vi "Get Devices In Family.vi"(8 "Error In":errorcluster, 11 "Device Family":T4) -> (0 "Error Out":errorcluster, 3 "Devices":string[](array[string]))   [LabVIEW 2013, in "LVH-LINX.lvlib"]
uses:
  <vilib>/LabVIEW Hacker/LINX/LVH-LINX.lvlib
  <vilib>/LabVIEW Hacker/LINX/Private/Type Defs/Device Family.ctl
  <vilib>/LabVIEW Hacker/LINX/Private/Type Defs/Devices - Digilent.ctl
  <vilib>/LabVIEW Hacker/LINX/Private/Type Defs/Devices - NI.ctl
  <vilib>/LabVIEW Hacker/LINX/Private/Type Defs/Devices - Arduino.ctl
panel:
  in  "Arduino Device":T1
  in  "NI Device":T2
  in  "Digilent Device":T3
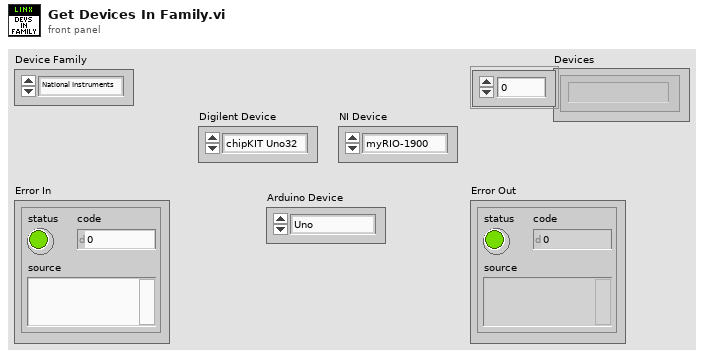
[diagram p1: front panel]
types:
  T1 = typedef "LVH-LINX.lvlib/Devices - Arduino.ctl" = enum16{"Uno", "Mega 2560", "Leonardo", "Due", "Yun", "Nano", "Pro Mini", "Pro", "Fio", "Mega1280"}
  T2 = typedef "LVH-LINX.lvlib/Devices - NI.ctl" = enum16{"myRIO-1900", "myRIO-1950"}
  T3 = typedef "LVH-LINX.lvlib/Devices - Digilent.ctl" = enum16{"chipKIT Uno32", "chipKIT uC32", "chipKIT Max32", "chipKIT WF32"}
  T4 = typedef "LVH-LINX.lvlib/Device Family.ctl" = enum8{"National Instruments", "Digilent", "Arduino"}
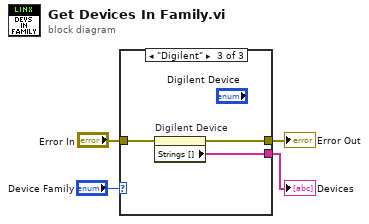
[diagram p0: block diagram]
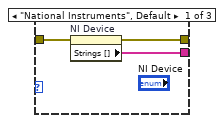
[diagram p2: hidden frame]
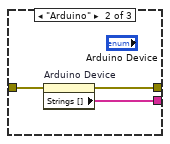
[diagram p3: hidden frame]
diagram:
  n1 = case shown="\"Digilent\"" "Device Family" {
    tunnel: "Error In" -> [w7 w9 w12]
    tunnel: [w5 w8 w13] -> w2
    tunnel: [w6 w10 w11] -> w1
    frame "National Instruments", Default {
      n2 = property on="NI Device" class="Enum (strict)"(error in=w7) -> (error out=w6:errorcluster, "Strings []"=w5:string[])  [unwired: 1 in, 1 out]
    }
    frame "Arduino" {
      n3 = property on="Arduino Device" class="Enum (strict)"(error in=w9) -> (error out=w10:errorcluster, "Strings []"=w8:string[])  [unwired: 1 in, 1 out]
    }
    frame "Digilent" {
      n4 = property on="Digilent Device" class="Enum (strict)"(error in=w12) -> (error out=w11:errorcluster, "Strings []"=w13:string[])  [unwired: 1 in, 1 out]
    }
  }
  "Error Out" <- w1
  "Devices" <- w2
